vi "Fetch ENA s-parameters.vi"() -> ()   [LabVIEW 2020]
uses:
  <vilib>/addons/HF Network Analysis/Controls/SnPDataType.ctl
  <instrlib>/Agilent ENA Series/Agilent ENA Series.lvlib
  <vilib>/addons/HF Network Analysis/NI_HFNetworkAnalysis.lvlib
panel:
  in  "SnP File Path":path
  out "XY Graph":T1(graph)
  out "X-Axis Data Measurement Points":dbl[](array[numeric])
  in  "VISA resource name":refnum<visa-resource-name>
  in  "error in (no error)":errorcluster
  out "Primary / Real":dbl[](array[numeric])
  out "Secondary / Imaginary":dbl[](array[numeric])
  in  "Source (0: Data)":u16(ring) items=["Data", "Memory"]
  in  "Correction (0: Data)":u16(ring) items=["Formatted", "Corrected"]
  in  "Channel (1)":i32=1
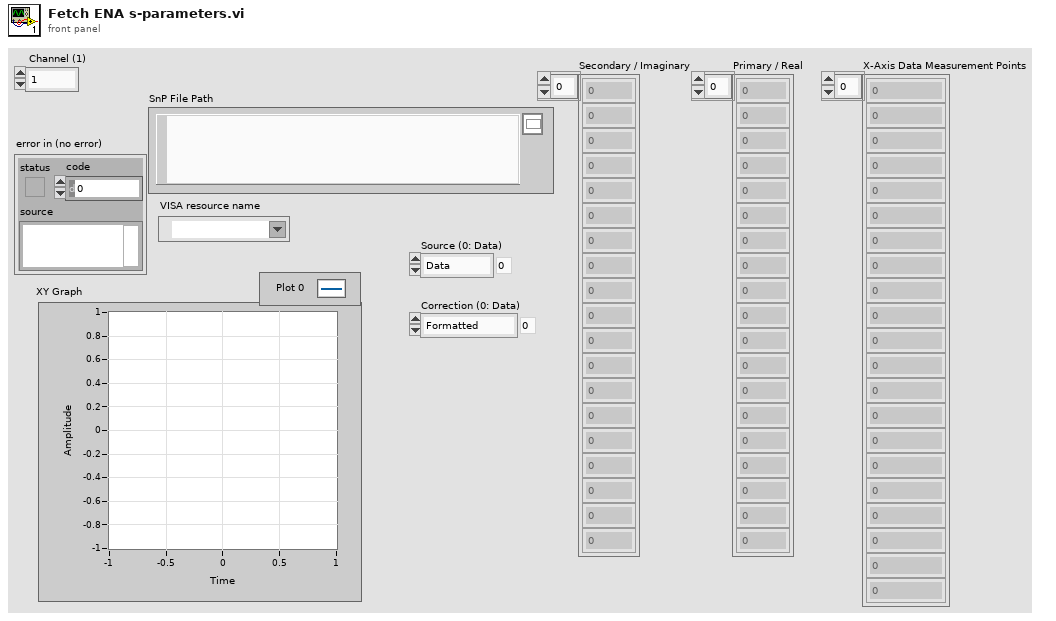
[diagram p1: front panel]
types:
  T1 = cluster{"Primary / Real":dbl[], "Secondary / Imaginary":dbl[]}
  T2 = typedef "NI_HFNetworkAnalysis.lvlib/SnPDataType.ctl" = enum16{"DB", "MA", "RI"}
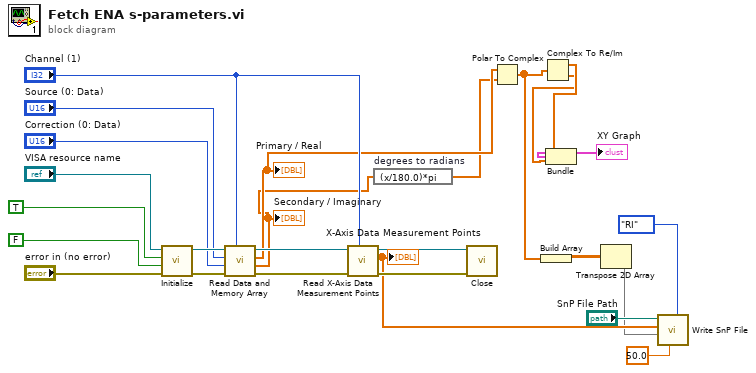
[diagram p0: block diagram]
diagram:
  n1 = call <instrlib>:"Initialize.vi"("error in (no error)"="error in (no error)", "Reset? (T: Yes)"=FALSE, "ID Query? (T: Yes)"=TRUE, "VISA resource name"="VISA resource name") -> ("error out"=w25:errorcluster, "VISA resource name out"=w26:refnum<visa-resource-name>)  [unwired: 6 in]
  n2 = call <instrlib>:"Read Data and Memory Array.vi"("Channel (1)"="Channel (1)", "error in (no error)"=w25, "Correction (0: Data)"="Correction (0: Data)", "Source (0: Data)"="Source (0: Data)", "VISA resource name"=w26) -> ("error out"=w17:errorcluster, "Secondary / Imaginary"=w11:dbl[], "Primary / Real"=w12:dbl[], "VISA resource name out"=w18:refnum<visa-resource-name>)  [unwired: 3 in]
  "Secondary / Imaginary" <- w11
  "Primary / Real" <- w12
  n3 = call <instrlib>:"Read X-Axis Data Measurement Points.vi"("Channel (1)"="Channel (1)", "error in (no error)"=w17, "VISA resource name"=w18) -> ("error out"=w15:errorcluster, "X-Axis Data Measurement Points"=w7:dbl[], "VISA resource name out"=w16:refnum<visa-resource-name>)  [unwired: 6 in]
  "X-Axis Data Measurement Points" <- w7
  n4 = expression code="(x/180.0)*pi" "degrees to radians"(w11) -> (w10:dbl[])
  n5 = call <instrlib>:"Close.vi"("error in (no error)"=w15, "VISA resource name"=w16) -> ()  [unwired: 9 in, 1 out]
  n6 = Polar To Complex(1:w10, 2:w12) -> (0:w4:cdb[])
  n7 = Build Array(w4) -> (w2:cdb[][])
  n8 = Complex To Re/Im(x + iy=w4) -> (x=w9:dbl[], y=w8:dbl[])
  n9 = Bundle(w9, w8) -> (→"XY Graph":cluster{dbl[], dbl[]})  [unwired: 1 in]
  n10 = Transpose 2D Array(2D array=w2) -> (transposed array=w1:cdb[][])
  n11 = call <vilib>:"Write SnP File.vi"("OutputDataType"=SnPDataType."RI", "Z0 (50 Ohm)"=50.0, "S-parameters"=w1, "Frequencies (Hz)"=w7, "SnP File Path"="SnP File Path") -> ()  [unwired: 6 in, 1 out]
